vi "Terminal-DriverSystem-Getter20150815.vi"(8 "error in (no error)":errorcluster caption="错误输入（无错误）", 11 "read operation timeout (ms)":i32=5000 caption="读操作超时（5000毫秒）") -> (0 "error out":errorcluster caption="错误输出", 2 "时间标识":timestamp, 3 "设备信息":T1)   [LabVIEW 2014]
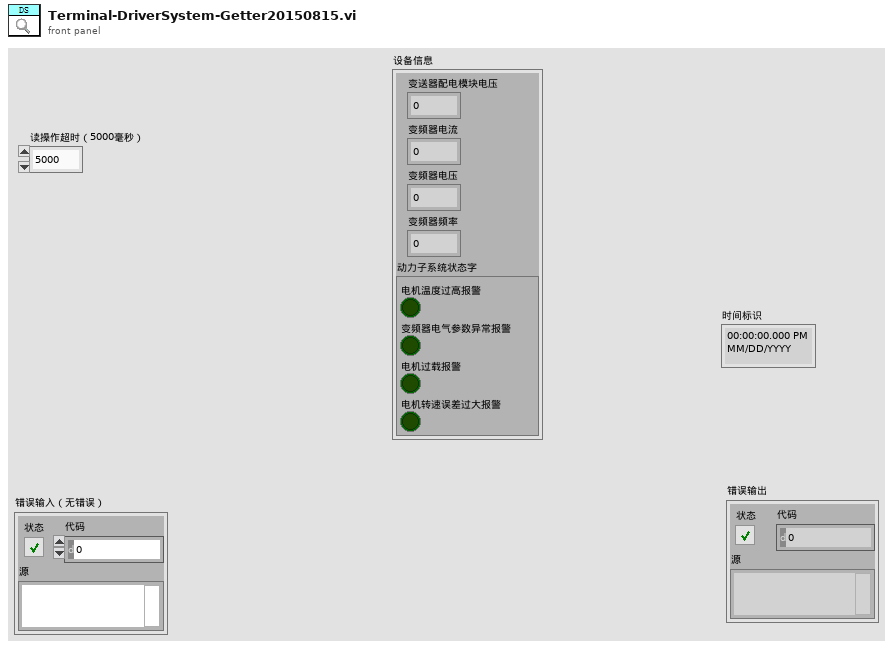
[diagram p1: front panel]
types:
  T1 = cluster{"变送器配电模块电压":u16, "变频器电流":u16, "变频器电压":u16, "变频器频率":u16, "动力子系统状态字":cluster{"电机温度过高报警":bool, "变频器电气参数异常报警":bool, "电机过载报警":bool, "电机转速误差过大报警":bool}}
  T2 = cluster{"电机温度过高报警":bool, "变频器电气参数异常报警":bool, "电机过载报警":bool, "电机转速误差过大报警":bool}
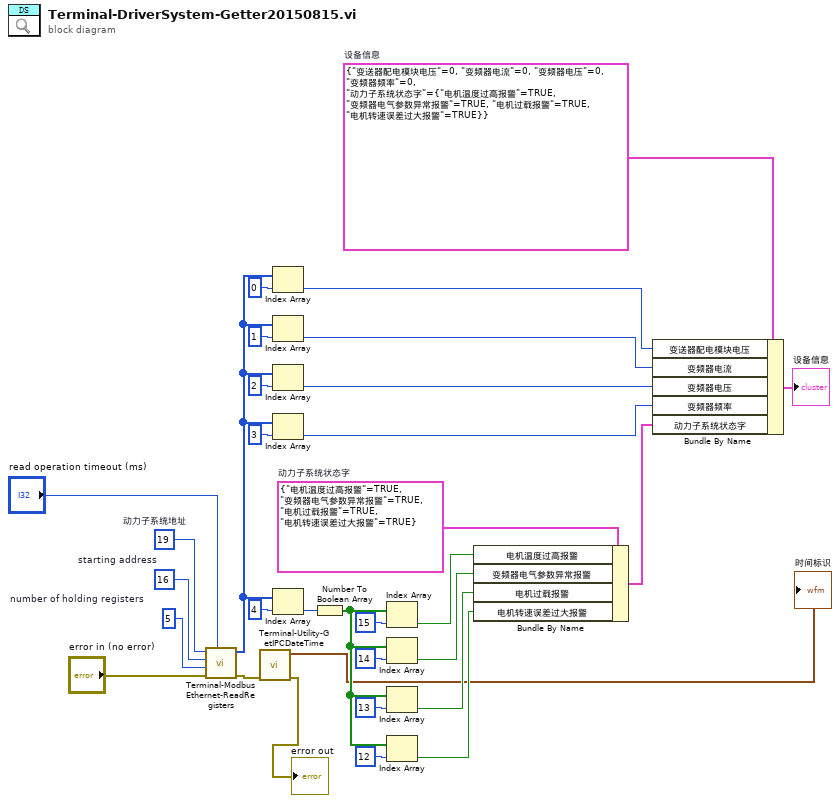
[diagram p0: block diagram]
diagram:
  w26 = T2 {"电机温度过高报警"=TRUE, "变频器电气参数异常报警"=TRUE, "电机过载报警"=TRUE, "电机转速误差过大报警"=TRUE}  # 动力子系统状态字
  w27 = T1 {"变送器配电模块电压"=0, "变频器电流"=0, "变频器电压"=0, "变频器频率"=0, "动力子系统状态字"={"电机温度过高报警"=TRUE, "变频器电气参数异常报警"=TRUE, "电机过载报警"=TRUE, "电机转速误差过大报警"=TRUE}}  # 设备信息
  w30 = u16 5  # number of holding registers
  w31 = u16 16  # starting address
  w32 = u8 19  # 动力子系统地址
  n1 = call "Terminal-ModbusEthernet-ReadRegisters.vi"("read operation timeout (ms)"="read operation timeout (ms)", "error in"="error in (no error)", "number of holding registers"=w30, "starting address"=w31, "unit ID"=w32) -> ("error out"=w3:errorcluster, "register values"=w15:u16[])  [unwired: 5 in]
  n2 = call "Terminal-Utility-GetIPCDateTime.vi"("error in (no error)"=w3) -> ("error out"=→"error out":errorcluster, "时间标识"=→"时间标识":timestamp)  [unwired: 9 in]
  n3 = Index Array(array=w15, index=0 ("索引")) -> (element=w23:u16)
  n4 = Index Array(array=w15, index=1 ("索引")) -> (element=w18:u16)
  n5 = Index Array(array=w15, index=2 ("索引")) -> (element=w17:u16)
  n6 = Index Array(array=w15, index=3 ("索引")) -> (element=w16:u16)
  n7 = Index Array(array=w15, index=4 ("索引")) -> (element=w14:u16)
  n8 = Number To Boolean Array(number=w14) -> (Boolean array=w9:bool[])
  n9 = Index Array(array=w9, index=15 ("索引")) -> (element=w8:bool)
  n10 = Index Array(array=w9, index=14 ("索引")) -> (element=w7:bool)
  n11 = Index Array(array=w9, index=13 ("索引")) -> (element=w6:bool)
  n12 = Index Array(array=w9, index=12 ("索引")) -> (element=w5:bool)
  n13 = Bundle By Name(cluster=w26, "电机温度过高报警"=w8, "变频器电气参数异常报警"=w7, "电机过载报警"=w6, "电机转速误差过大报警"=w5) -> (w25:T2)
  n14 = Bundle By Name(cluster=w27, "变送器配电模块电压"=w23, "变频器电流"=w18, "变频器电压"=w17, "变频器频率"=w16, "动力子系统状态字"=w25) -> (→"设备信息":T1)
